vi "CCIP.vi"(0 "Camera angle":dbl, 1 "zAvit":dbl, 3 "Processed Image":T2(plugin-control), 5 "Camera off set":dbl, 7 "Distance (from camera to target)":dbl, 9 "Compliting angle to 180":dbl, 12 "X center":dbl, 13 "Y center":dbl, 14 "Particle Scores":T1) -> (8 "Processed Image + aim markings":T2(plugin-control), 10 "Height from cannon":dbl, 15 "Distance from cannon":dbl)   [LabVIEW 2012]
panel:
  in  "Convert Direction":u16(ring) items=["Nums to Pixels", "Pixel to Nums"]
  # "Shoot varubalse"
  # "Off set calculating"
  # "Drawing"
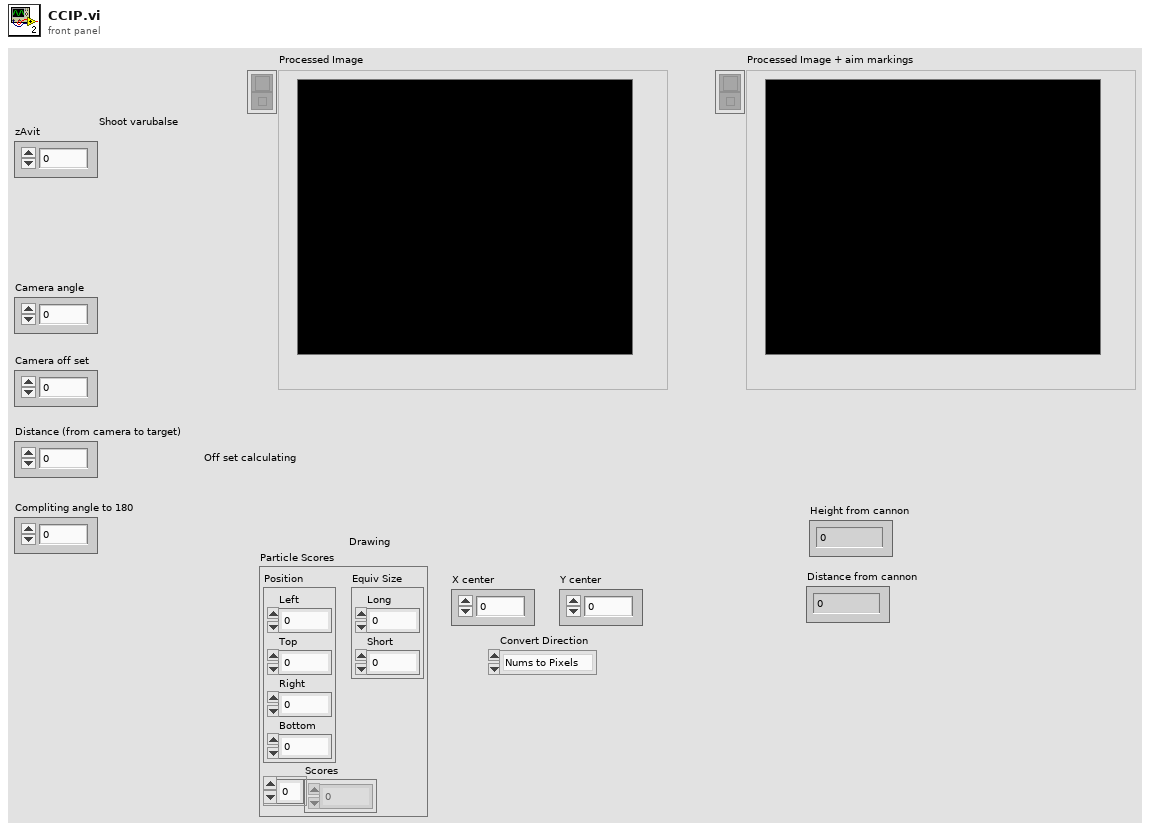
[diagram p1: front panel]
types:
  T1 = cluster{"Position":cluster{"Left":dbl, "Top":dbl, "Right":dbl, "Bottom":dbl}, "Scores":dbl[], "Equiv Size":cluster{"Long":dbl, "Short":dbl}}
  T2 = typedef "IMAQ Image.ctl" = refnum<image>
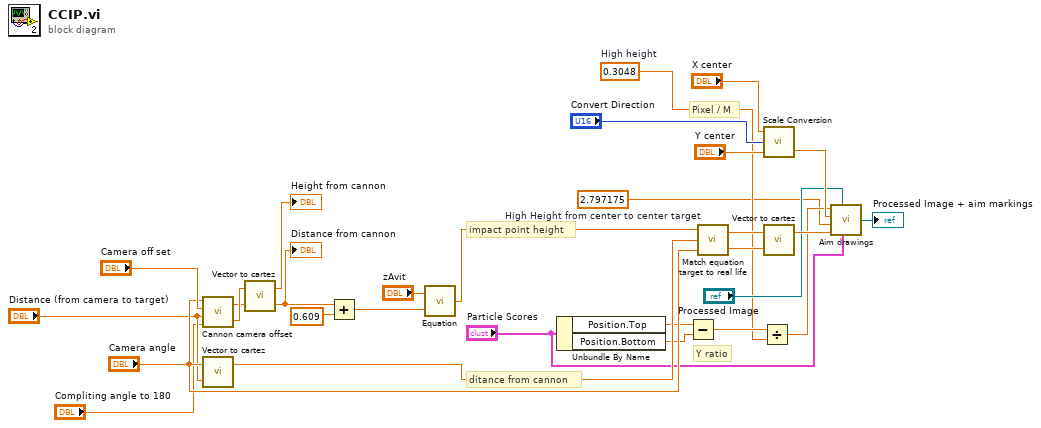
[diagram p0: block diagram]
diagram:
  w8 = 0.3048  # High height
  w7 = 2.797175  # High Height from center to center target
  # "Pixel / M"
  # "impact point height"
  # "ditance from cannon"
  # "Y ratio"
  n1 = call "Cannon camera offset.vi"("Compliting angle to 180"="Compliting angle to 180", "Distance (from camera)"="Distance (from camera to target)", "Offset (from center axis to camera lens)"="Camera off set", "Camera angle"="Camera angle") -> ("Angle (from cannon to target)"=w25:dbl, "Distance from cannon"=w3:dbl)
  n2 = call "Vector to cartez.vi"("Vector"="Distance (from camera to target)", "Angle [deg]"="Camera angle") -> ("Height"=w24:dbl)  [unwired: 1 out]
  n3 = call "Vector to cartez.vi"("Vector"=w3, "Angle [deg]"=w25) -> ("Length"=w2:dbl, "Height"=→"Height from cannon":dbl)
  "Distance from cannon" <- w2
  n4 = Add(x=w2, y=0.609) -> (x+y=w4:dbl)
  n5 = call "Equation.vi"("Distance"=w4, "zAvit"="zAvit") -> ("Calculated Height"=w6:dbl)
  n6 = Unbundle By Name("Particle Scores") -> ("Position.Top"=w12:dbl, "Position.Bottom"=w11:dbl)
  n7 = Subtract(x=w12, y=w11) -> (x-y=w10:dbl)
  n8 = call "Match equation target to real life.vi"("Camera angle"="Camera angle", "Height from camera"=w24, "Calculated height"=w6) -> ("Distance from Camera"=w20:dbl, "Angle on Camera"=w21:dbl)
  n9 = Divide(x=w10, y=w8) -> (x/y=w16:dbl)
  n10 = call "Scale Conversion.vi"("y in"="Y center", "Convert Direction"="Convert Direction", "x in"="X center") -> ("y out"=w18:dbl)  [unwired: 1 out]
  n11 = call "Vector to cartez.vi"("Vector"=w20, "Angle [deg]"=w21) -> ("Height"=w17:dbl)  [unwired: 1 out]
  n12 = call "Aim drawings.vi"("Particle Scores"="Particle Scores", "Processed Image"="Processed Image", "Calculated height [m]"=w17, "Center target position real life height [m]"=w7, "Center target position Y"=w18, "Y ratio"=w16) -> ("Processed Image + aim markings"=→"Processed Image + aim markings":T2)
